vi "Convert_allChannelProperties_to_JSON.vi"(8 "error in (no error)":errorcluster, 11 "allChannelProperties":T1 {"channel" min=1 max=8 step=1}) -> (0 "error out":errorcluster, 3 "<JSON>":string)   [LabVIEW 2019, in "Inst.Krohn-Hite-7008.lvclass"]
uses:
  Inst.Krohn-Hite-7008.lvclass
  KH7008/typedefs/allChannelProperties--Array.ctl
  KH7008/typedefs/channelProperties--Cluster.ctl
  KH7008/typedefs/channel--numeric.ctl
  KH7008/typedefs/gain--enum.ctl
  KH7008/typedefs/Input--Enum.ctl
  KH7008/typedefs/shunt--enum.ctl
  KH7008/typedefs/couple--Enum.ctl
  KH7008/typedefs/Filter--Enum.ctl
  Typedefs/getAllChannelsDatabase--Cluster.ctl
  3cd287df-e11a-49e5-8b51-e9e2427607d6.vi
  <vilib>/JDP Science/JSONtext/Variant to JSON Text.vi
  <vilib>/JDP Science/JSONtext/LVClass Serializer/JSONtext LVClass Serializer.lvclass
  KH7008/KH7008.lvlib
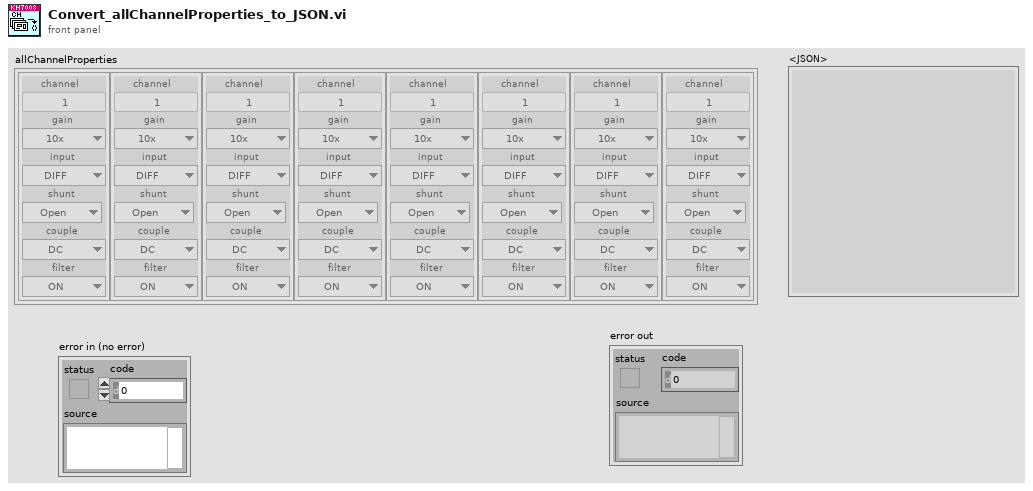
[diagram p1: front panel]
types:
  T1 = typedef "KH7008.lvlib/allChannelProperties--Array.ctl" = T2[]
  T2 = typedef "KH7008.lvlib/channelProperties--Cluster.ctl" = cluster{"channel":T3, "gain":T4, "input":T5, "shunt":T6, "couple":T7, "filter":T8}
  T3 = typedef "KH7008.lvlib/channel--numeric.ctl" = u16
  T4 = typedef "KH7008.lvlib/gain--enum.ctl" = enum16{"1x", "10x", "100x", "1000x"}
  T5 = typedef "KH7008.lvlib/input--enum.ctl" = enum16{"OFF", "SE+", "SE-", "DIFF"}
  T6 = typedef "KH7008.lvlib/shunt--enum.ctl" = enum16{"Open", "50", "500", "5k", "50k", "10M"}
  T7 = typedef "KH7008.lvlib/couple--enum.ctl" = enum16{"AC", "DC"}
  T8 = typedef "KH7008.lvlib/filter--enum.ctl" = enum16{"OFF", "ON"}
  T9 = typedef "Inst.Krohn-Hite-7008.lvclass/getAllChannelsDatabase--Cluster.ctl" = cluster{"channel":u32, "gain":u32, "input":string, "shunt":u32, "couple":string, "filter":string}
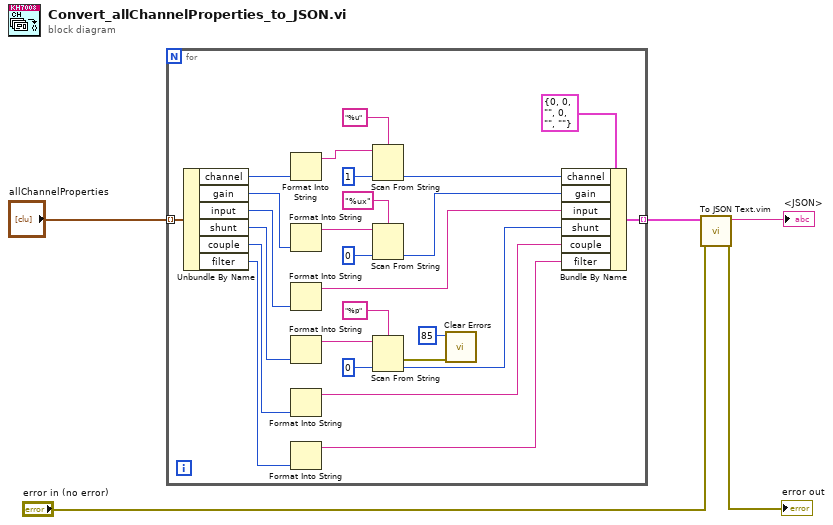
[diagram p0: block diagram]
diagram:
  n1 = for {
    tunnel: "allChannelProperties" -> [w31] mode=indexing
    tunnel: [w29] -> w5 mode=indexing
    n2 = Unbundle By Name(w31) -> ("channel"=w7:T3, "gain"=w6:T4, "input"=w8:T5, "shunt"=w9:T6, "couple"=w10:T7, "filter"=w11:T8)
    n3 = Format Into String(w7) -> (resulting string=w22:string)  [unwired: 3 in, 1 out]
    n4 = Format Into String(w6) -> (resulting string=w24:string)  [unwired: 3 in, 1 out]
    n5 = Format Into String(w8) -> (resulting string=w28:string)  [unwired: 3 in, 1 out]
    n6 = Format Into String(w9) -> (resulting string=w16:string)  [unwired: 3 in, 1 out]
    n7 = Format Into String(w10) -> (resulting string=w26:string)  [unwired: 3 in, 1 out]
    n8 = Format Into String(w11) -> (resulting string=w27:string)  [unwired: 3 in, 1 out]
    n9 = Scan From String(format string="%u", input string=w22, default 1=u32 1 ("default value 1")) -> (output 1=w20:u32)  [unwired: 2 in, 3 out]
    n10 = Scan From String(format string="%ux", input string=w24, default 1=u32 0 ("default value 1")) -> (output 1=w15:u32)  [unwired: 2 in, 3 out]
    n11 = Scan From String(format string="%p", input string=w16, default 1=u32 0 ("default value 1")) -> (error out=w12:errorcluster, output 1=w14:u32)  [unwired: 2 in, 2 out]
    n12 = call <vilib>:"Clear Errors.vi"("error in (no error)"=w12, "specific error code to clear (0: all)"=85) -> ()  [unwired: 4 in, 2 out]
    n13 = Bundle By Name(cluster=T9 {"channel"=0, "gain"=0, "input"="", "shunt"=0, "couple"="", "filter"=""} ("getAllChannelsResponse"), "channel"=w20, "gain"=w15, "input"=w28, "shunt"=w14, "couple"=w26, "filter"=w27) -> (w29:T9)
  }
  n14 = call "To JSON Text.vim"("error in (no error)"="error in (no error)", "Anything"=w5) -> ("error out"=→"error out":errorcluster, "<JSON>"=→"<JSON>":string)  [unwired: 8 in]
